vi "LuaVIEW Close.vi"(5 "LuaVIEW reference":T1, 11 "error in (no error)":errorcluster) -> (15 "dup error":errorcluster)   [LabVIEW 2013]
doc: "Closes a LuaVIEW reference as returned by \"LuaVIEW Open\". This closes the Lua state associated with the references and decrements the function registry usage count. When the usage count reaches zero, the function registry is cleaned up.\n\nThis function executes irrespective of the input error so that the reference is closed and registry use count is decremented even when one of the preceeding chained VIs failed. It does not execute when a default (nil) reference is provided, as returned by a failed \"LuaVIEW Open\" or an uninitialized shift register. Do not close or otherwise use an already closed reference. Though LuaVIEW performs checks to avoid operating on closed states, this is only 99.999% safe."
uses:
  typedefs/t_LuaVIEW Reference.ctl
  typedefs/t_LuaVIEW CIN Spinlocked Actions.ctl
  typedefs/et_LuaVIEW CIN Actions.ctl
  glb_LuaVIEW Configuration Globals.vi
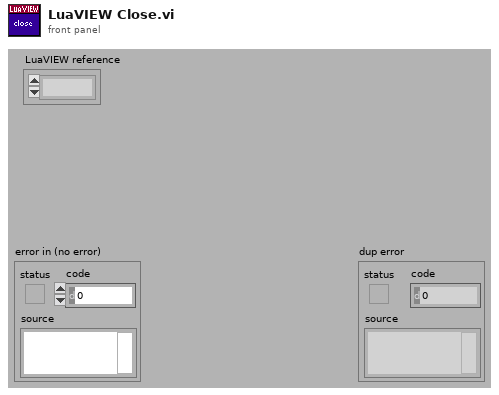
[diagram p1: front panel]
types:
  T1 = typedef "t_LuaVIEW Reference.ctl" = refnum<k1>
  T2 = typedef "t_LuaVIEW CIN Spinlocked Actions.ctl" = enum16{"totals", "taskcount", "open", "registerpublic", "registerexport", "revokeexports", "unregnextpublic", "usepublic", "pollexport", "close", "startyieldtest", "endyieldtest", "pollprintbuffer"}
  T3 = typedef "et_LuaVIEW CIN Actions.ctl" = enum16{"checksynopsis", "_open", "_registerpublic", "_registerexport", "__never_an_error_result_ns", "luaversion", "cinversion", "_totals", "_taskcount", "pathological", "_unregnextpublic", "registryusecount", "__per_state_actions", "regsetprivate", "regsetindex", "regsetmodule", "_revokeexports", "_usepublic", "prepare", "compile", "execute", "call", "unregstaterefs", "_close", "pullboolean", "pullnumber", "pullI8", "pullU8", "pullI16", "pullU16", "pullI32", "pullU32", "pullobject", "pullrefnum", "pullstring", "pullflat", "pushflat", "pushobject", "getattribute", "setattribute", "stacktostring", "_startyieldtest", "_endyieldtest", "_pollprintbuffer", "__never_an_error_result_ps", "_pollexport", "setclone", "forcecleanup", "gettop", "clearstack", "insert", "pushboolean", "pushnumber", "pushrefnum", "pushstring", "pushnil", "pushvalue", "gettaskref", "settaskref"}
  T4 = typedef "et_LuaVIEW CIN Results.ctl" = enum16{"OK", "error", "main", "call", "clonecall", "modulecall", "exportcall", "index", "yield"}
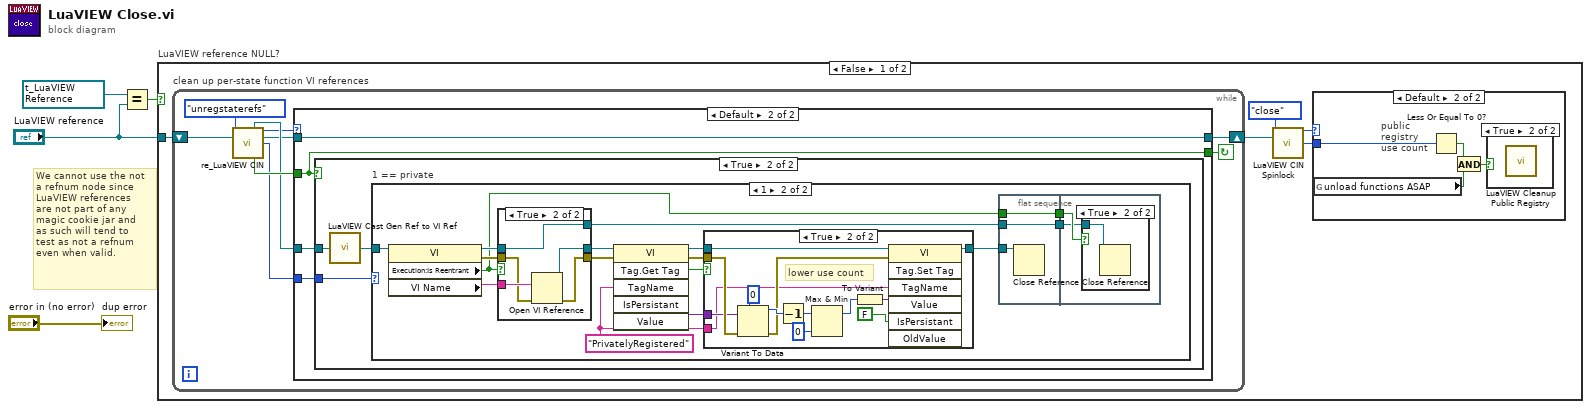
[diagram p0: block diagram]
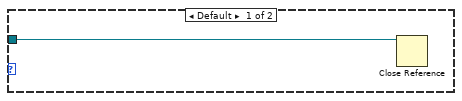
[diagram p6: hidden frame]
diagram:
  w2 = T1 refnum items=["LuaVIEW"] ("LuaVIEW reference")
  # "We cannot use the not\na refnum node since\nLuaVIEW references\nare not part of any\nmagic cookie jar and\nas such will tend to\ntest as not a refnum\neven when valid."
  n1 = Equal?(x=w2, y="LuaVIEW reference") -> (x = y?=w3:bool)
  n2 = case "LuaVIEW reference NULL?" shown="False" w3 {
    tunnel: "LuaVIEW reference" -> [w8 _]
    frame False {
      n3 = while "clean up per-state function VI references" {
        shift-right: [w16] -> w7
        shift-left: w8 -> [w22]
        stop <- w14 continue-if-true
        n4 = call "re_LuaVIEW CIN.vi"("action"=et_LuaVIEW_CIN_Actions."unregstaterefs", "LuaVIEW reference in"=w22) -> ("refnum out"=w19:refnum<vi>, "result"=w15:T4, "LuaVIEW reference out"=w17:T1, "index out"=w18:i32, "boolean out"=w20:bool)  [unwired: 7 in, 2 out]
        n5 = case shown="Default" w15 {
          tunnel: w20 -> [_ w24]
          tunnel: w19 -> [_ w27]
          tunnel: w18 -> [_ w26]
          tunnel: w17 -> [w23 w25]
          tunnel: [w23 w25] -> w16
          tunnel: [_ w24] -> w14
          frame "error" {
            # "dead or invalid reference"
          }
          frame Default {
            n6 = case shown="True" w24 {
              tunnel: w27 -> [_ w30]
              tunnel: w26 -> [_ w28]
              frame False {
              }
              frame True {
                n7 = call "LuaVIEW Cast Gen Ref to VI Ref.vi"("refnum in"=w30) -> ("refnum out"=w29:refnum<vi>)  [unwired: 14 in]
                n8 = case "1 == private" shown="1" w28 {
                  tunnel: w29 -> [w31 w42]
                  frame Default {
                    n9 = Close Reference(reference=w31) -> ()  [unwired: 1 in, 1 out]
                  }
                  frame 1 {
                    w43 = "PrivatelyRegistered"
                    n10 = property class="VI"(reference=w42) -> (reference out=w36:refnum<vi>, error out=w40:errorcluster, "Execution:Is Reentrant"=w32:bool, "VI Name"=w41:string)  [unwired: 1 in]
                    n11 = case shown="True" w32 {
                      tunnel: w41 -> [_ w60]
                      tunnel: w40 -> [w55 w59]
                      tunnel: [w55 w58] -> w39
                      tunnel: [w54 w57] -> w38
                      tunnel: w36 -> [w54 w56]
                      tunnel: [_ w56] -> w34
                      frame False {
                      }
                      frame True {
                        n12 = Open VI Reference(vi path=w60, error in (no error)=w59) -> (vi reference=w57:refnum<vi>, error out=w58:errorcluster)  [unwired: 4 in]
                      }
                    }
                    n13 = invoke class="VI" method="Tag.Get Tag"(reference=w38, error in=w39, "TagName"=w43) -> (reference out=w44:refnum<vi>, error out=w45:errorcluster, "GetTag"=w47:bool, "Value"=w46:variant)  [unwired: 3 in, 2 out]
                    n14 = case shown="True" w47 {
                      tunnel: w46 -> [_ w72]
                      tunnel: w45 -> [_ w73]
                      tunnel: w44 -> [w61 w65]
                      tunnel: [w61 w63] -> w37
                      tunnel: w43 -> [_ w62]
                      frame False {
                      }
                      frame True {
                        # "lower use count"
                        n15 = Variant To Data(error in=w73, type=0, Variant=w72) -> (data=w71:i32, error out=w64:errorcluster)
                        n16 = Decrement(x=w71) -> (x-1=w68:i32)
                        n17 = Max & Min(x=w68, y=0) -> (max(x,y)=w66:i32)  [unwired: 1 out]
                        n18 = To Variant(anything=w66) -> (Variant=w70:variant)
                        n19 = invoke class="VI" method="Tag.Set Tag"(reference=w65, error in=w64, "TagName"=w62, "Value"=w70, "IsPersistant"=FALSE) -> (reference out=w63:refnum<vi>)  [unwired: 2 in, 6 out]
                      }
                    }
                    n20 = flat-sequence {
                      tunnel: w37 -> [w50]
                      tunnel: [w49] -> w35
                      tunnel: w34 -> [w49]
                      tunnel: [w48] -> w33
                      tunnel: w32 -> [w48]
                      tunnel: w35 -> [w51]
                      tunnel: w33 -> [w52]
                      frame #0 {
                        n21 = Close Reference(reference=w50) -> ()  [unwired: 1 in, 1 out]
                      }
                      frame #1 {
                        n22 = case shown="True" w52 {
                          tunnel: w51 -> [_ w53]
                          frame False {
                          }
                          frame True {
                            n23 = Close Reference(reference=w53) -> ()  [unwired: 1 in, 1 out]
                          }
                        }
                      }
                    }
                  }
                }
              }
            }
          }
        }
      }
      n24 = call "LuaVIEW CIN Spinlock.vi"("action"=t_LuaVIEW_CIN_Spinlocked_Actions."close", "LuaVIEW reference in"=w7) -> ("result"=w5:T4, "index out"=w6:i32)  [unwired: 7 in, 5 out]
      n25 = case shown="Default" w5 {
        tunnel: w6 -> [_ w13]
        frame "error" {
          # "dead or invalid reference"
        }
        frame Default {
          # "public\nregistry\nuse count"
          n26 = global read "glb_LuaVIEW Configuration Globals.vi" "unload functions ASAP"() -> (w11:bool)
          n27 = Less Or Equal To 0?(x=w13) -> (x <= 0?=w12:bool)
          n28 = And(x=w12, y=w11) -> (x .and. y?=w10:bool)
          n29 = case shown="True" w10 {
            frame False {
            }
            frame True {
              n30 = call "LuaVIEW Cleanup Public Registry.vi"() -> ()  [unwired: 15 in, 1 out]
            }
          }
        }
      }
    }
    frame True {
    }
  }
  "dup error" <- "error in (no error)"
